vi "SetWindowIcon.vi"(8 "No Error":errorcluster, 10 "Icon [SDL_Surface *]":i64 format="%.0x", 11 "Window [SDL_Window *]":i64 format="%.0x") -> (0 "Error Out":errorcluster)   [LabVIEW 2024, in "SDL3.lvlib" / "Video.lvlib"]
doc: "<B>Summary</B>\nSet the icon for a window.\n\n<B>Remarks</B>\nIf this function is passed a surface with alternate representations, the surface will be interpreted as the content to be used for 100% display scale, and the alternate representations will be used for high DPI situations. For example, if the original surface is 32x32, then on a 2x macOS display or 200% display scale on Windows, a 64x64 version of the image will be used, if available. If a matching version of the image isn't available, the closest larger size image will be downscaled to the appropriate size and be used instead, if available. Otherwise, the closest smaller image will be upscaled and be used instead."
uses:
  Video.lvlib
  Error/Error.lvlib
  Lib/SDL3-32.dll
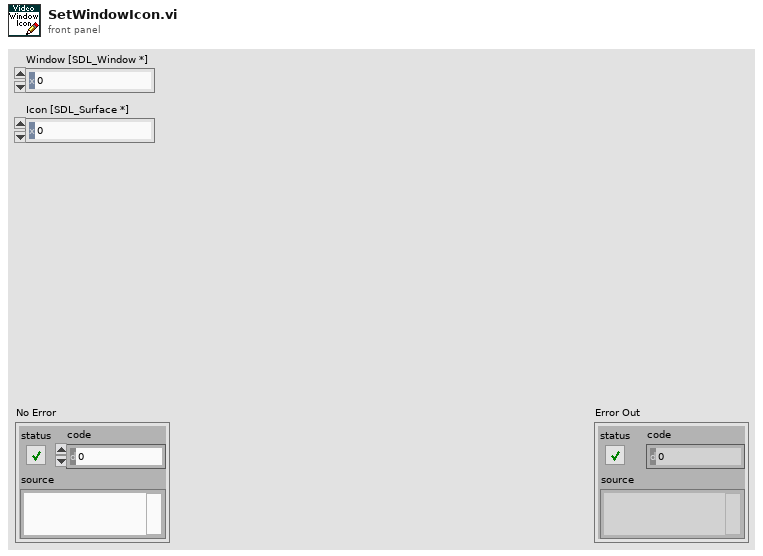
[diagram p1: front panel]
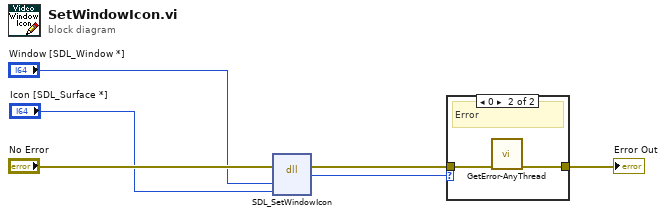
[diagram p0: block diagram]
diagram:
  n1 = dll-call lib="C:/Users/Thomas/Documents/Projects/LV-SDL3/Lib/SDL3-*.*" fn="SDL_SetWindowIcon"(error in="No Error", "window"="Window [SDL_Window *]", "icon"="Icon [SDL_Surface *]") -> (error out=w3:errorcluster, "return type"=w2:i32)  [unwired: 4 in, 1 out]
  n2 = case shown="0" w2 {
    tunnel: w3 -> [w7 w9]
    tunnel: [w7 w8] -> w5
    frame Default {
      # "Ok"
    }
    frame 0 {
      # "Error"
      n3 = call "GetError-AnyThread.vi"("No Error"=w9) -> ("Error Out"=w8:errorcluster)  [unwired: 10 in]
    }
  }
  "Error Out" <- w5
